vi "版本判断.vi"(7 "Extern":bool, 11 "固件版本号":string) -> (3 "仪器版本":T1)   [LabVIEW 2016, in "斯坦道总氮.lvlib"]
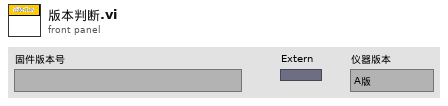
[diagram p1: front panel]
types:
  T1 = typedef "SingleStepTestV3.lvlib/SingleStepTestV3.lvclass/仪器版本.ctl" = enum16{"A版", "B版", "A1版"}
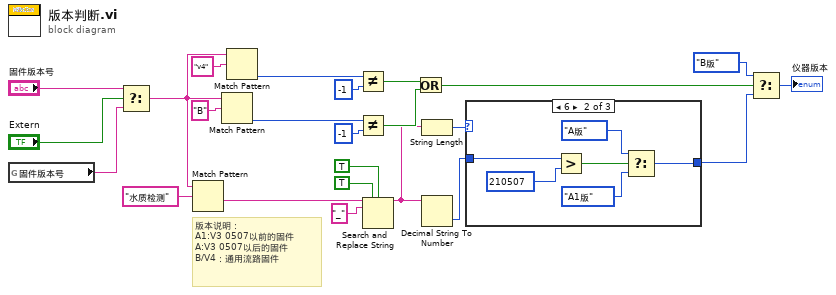
[diagram p0: block diagram]
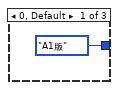
[diagram p2: hidden frame]
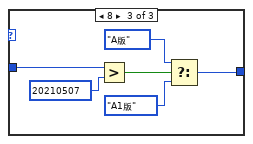
[diagram p3: hidden frame]
diagram:
  # "版本说明：\nA1:V3 0507以前的固件\nA:V3 0507以后的固件\nB/V4：通用流路固件"
  n1 = global read "VAR总磷总氮全局变量.vi" "固件版本号"() -> (w7:string)
  n2 = Select(t="固件版本号", s="Extern", f=w7) -> (s? t:f=w5:string)
  n3 = Match Pattern(string=w5, regular expression="水质检测" ("正则表达式")) -> (after substring=w17:string)  [unwired: 1 in, 3 out]
  n4 = Match Pattern(string=w5, regular expression="B" ("正则表达式")) -> (offset past match=w20:i32)  [unwired: 1 in, 3 out]
  n5 = Match Pattern(string=w5, regular expression="v4" ("正则表达式")) -> (offset past match=w3:i32)  [unwired: 1 in, 3 out]
  n6 = Not Equal?(x=w3, y=-1) -> (x != y?=w1:bool)
  n7 = Not Equal?(x=w20, y=-1) -> (x != y?=w22:bool)
  n8 = Search and Replace String(replace all?=TRUE ("替换全部？(F)"), case sensitive?=TRUE ("忽略大小写？(F)"), input string=w17, search string="_" ("搜索字符串")) -> (result string=w12:string)  [unwired: 4 in, 3 out]
  n9 = Or(x=w1, y=w22) -> (x .or. y?=w2:bool)
  n10 = String Length(string=w12) -> (length=w13:i32)
  n11 = Decimal String To Number(string=w12) -> (number=w11:i32)  [unwired: 2 in, 1 out]
  n12 = case shown="6" w13 {
    tunnel: [仪器版本."A1版" ("仪器版本") w27 w33] -> w10
    tunnel: w11 -> [_ w26 w32]
    frame 0, Default {
    }
    frame 6 {
      n13 = Greater?(x=w26, y=210507) -> (0:w30:bool)
      n14 = Select(t=仪器版本."A版" ("仪器版本"), s=w30, f=仪器版本."A1版" ("仪器版本")) -> (s? t:f=w27:T1)
    }
    frame 8 {
      n15 = Greater?(x=w32, y=20210507) -> (0:w36:bool)
      n16 = Select(t=仪器版本."A版" ("仪器版本"), s=w36, f=仪器版本."A1版" ("仪器版本")) -> (s? t:f=w33:T1)
    }
  }
  n17 = Select(t=仪器版本."B版" ("仪器版本"), s=w2, f=w10) -> (s? t:f=→"仪器版本":T1)
